vi "GET Z Scan Size.vi"() -> (0 "Z Scan Size":dbl)   [LabVIEW 2013]
uses:
  Action.ctl
  Experimental Parameters FGV Selector.ctl
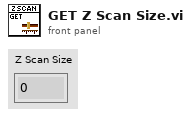
[diagram p1: front panel]
types:
  T1 = typedef "Experimental Parameters FGV Selector.ctl" = enum16{"Number of Samples", "Ramp Rate", "Z Scan Size"}
  T2 = typedef "Action.ctl" = enum16{"GET", "PUT", "DELETE"}
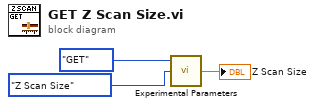
[diagram p0: block diagram]
diagram:
  n1 = call "Experimental Parameters.vi"("Experimental Parameters FGV Selector"=Experimental_Parameters_FGV_Selector."Z Scan Size", "Action"=Action."GET") -> ("Output"=→"Z Scan Size":dbl)  [unwired: 1 in]
